vi "SUB_COM_W_CharByCharNoCarrige_HEX_NOREAD.vi"(2 "cmd string":string, 3 "duplicate VISA resource name":refnum<visa-resource-name>) -> (1 "VISA resource OUT":refnum<visa-resource-name>)   [LabVIEW 2011]
panel:
  out "LOOP":i32
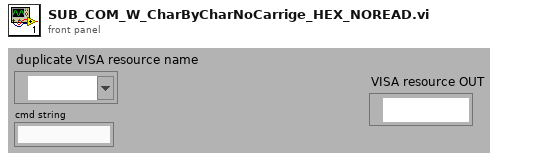
[diagram p1: front panel]
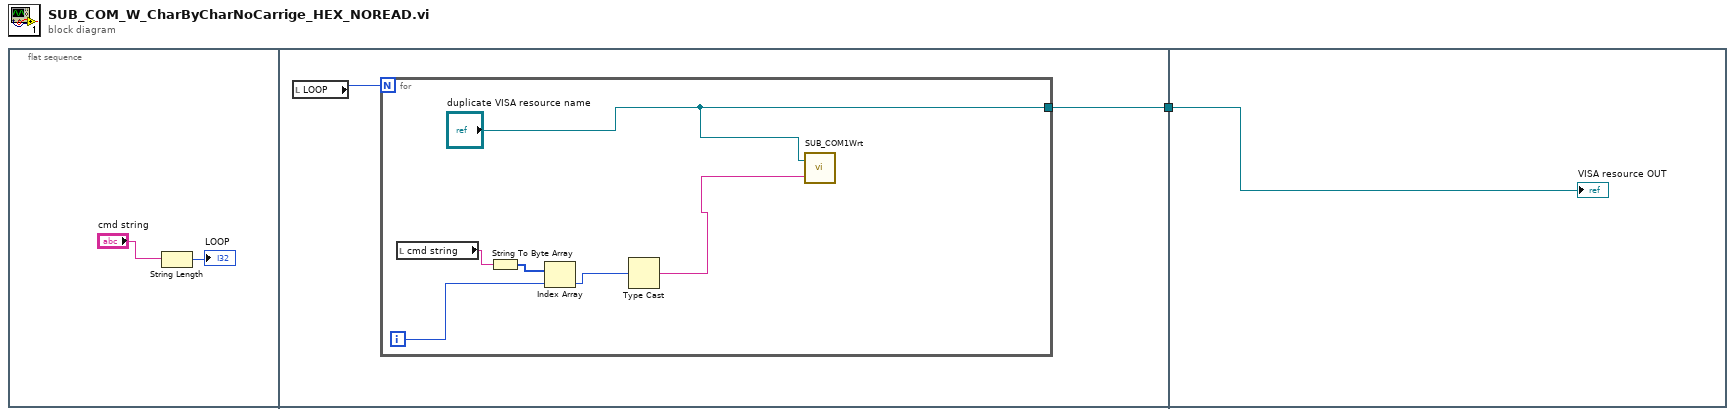
[diagram p0: block diagram]
diagram:
  n1 = flat-sequence {
    tunnel: [w4] -> w1
    tunnel: w1 -> [w12]
    frame #0 {
      n2 = String Length(string="cmd string") -> (length=→"LOOP":i32)
    }
    frame #1 {
      n3 = local read "LOOP"() -> (w5:i32)
      n4 = for {
        N: w5 -> [_]
        tunnel: ["duplicate VISA resource name"] -> w4
        i -> [w9]
        n5 = local read "cmd string"() -> (w11:string)
        n6 = String To Byte Array(string=w11) -> (unsigned byte array=w10:u8[])
        n7 = Index Array(array=w10, index=w9) -> (element=w8:u8)
        n8 = Type Cast(x=w8) -> (*(type *) &x=w7:string)  [unwired: 1 in]
        n9 = call "SUB_COM1Wrt.vi"("VISA resource name"="duplicate VISA resource name", "write buffer"=w7) -> ()  [unwired: 3 out]
      }
    }
    frame #2 {
      "VISA resource OUT" <- w12
    }
  }
